vi "GetAttributes.vi"(0 "ClassReaderGOOP300 in":refnum<class "ClassReaderGOOP300.lvclass">, 1 "OnlyGetReference":bool, 5 "error in (no error)":errorcluster) -> (14 "ClassReaderGOOP300 out":refnum<class "ClassReaderGOOP300.lvclass">, 15 "ObjectAttributes":T1[](array[typedef])=[{"name"="MyU8", "type"=enum."UINT8", "dimension"=0, "typeName"="", "typePath"=path "", "visibility"=enum."Protected"}, {"name"="MyStrArray", "type"=enum."STRING", "dimension"=1, "typeName"="", "typePath"=path "", "visibility"=enum."Protected"}], 16 "ClassAttributes":T1[](array[typedef])=[{"name"="MyU8", "type"=enum."UINT8", "dimension"=0, "typeName"="", "typePath"=path "", "visibility"=enum."Protected"}, {"name"="MyStrArray", "type"=enum."STRING", "dimension"=1, "typeName"="", "typePath"=path "", "visibility"=enum."Protected"}], 17 "ObjectAttributeReference":refnum<vi>, 18 "ClassAttributeReference":refnum<vi>, 19 "error out":errorcluster)   [LabVIEW 2012, in "ClassReaderGOOP300.lvclass"]
uses:
  <resource>/Framework/Providers/Open_GDS/ClassProviders/Provider_EndevoGOOP300/ClassReaderGOOP300_class/ClassReaderGOOP300.lvclass
  <resource>/Framework/Providers/Open_GDS/UML/ReversedEngineering/ReversedEngineering AttributeInfoType.ctl
  <resource>/Framework/Providers/Open_GDS/ClassProviders/Common/CommonVIs/CommonVIs_AttributeDataType.ctl
  <resource>/Framework/Providers/Open_GDS/UML/UMLEditor/UMLEditor_VisibilityType.ctl
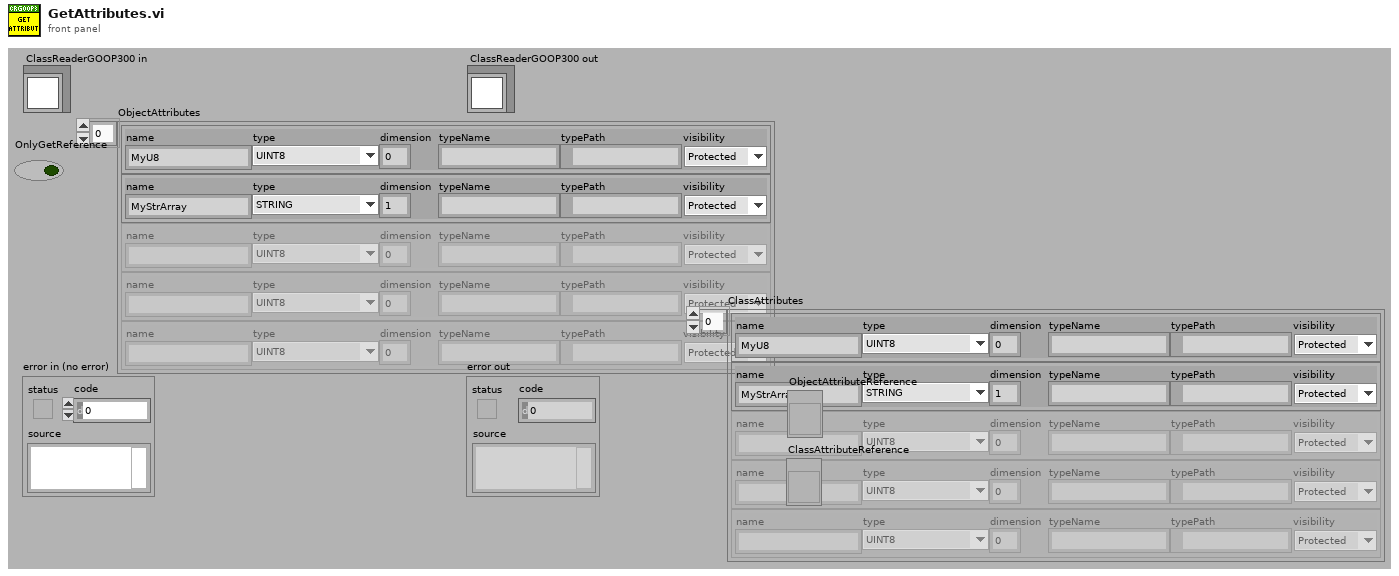
[diagram p1: front panel]
types:
  T1 = typedef "ReversedEngineering AttributeInfoType.ctl" = cluster{"name":string, "type":T2, "dimension":i32, "typeName":string, "typePath":path, "visibility":T3}
  T2 = typedef "CommonVIs_AttributeDataType.ctl" = enum16{"UINT8", "INT8", "UINT16", "INT16", "UINT32", "INT32", "UINT64", "INT64", "SGL", "DBL", "EXT", "CSG", "CDB", "CXT", "TimeStamp", "STRING", "PATH", "BOOL", "ENUM", "RefNum", "VIRefNum", "LabVIEW Class", "Cluster", "Variant", "TypeDef", "Waveform", "LabVIEW Object", "Other", "void"}
  T3 = typedef "UMLEditor_VisibilityType.ctl" = enum16{"Public", "Private", "Protected"}
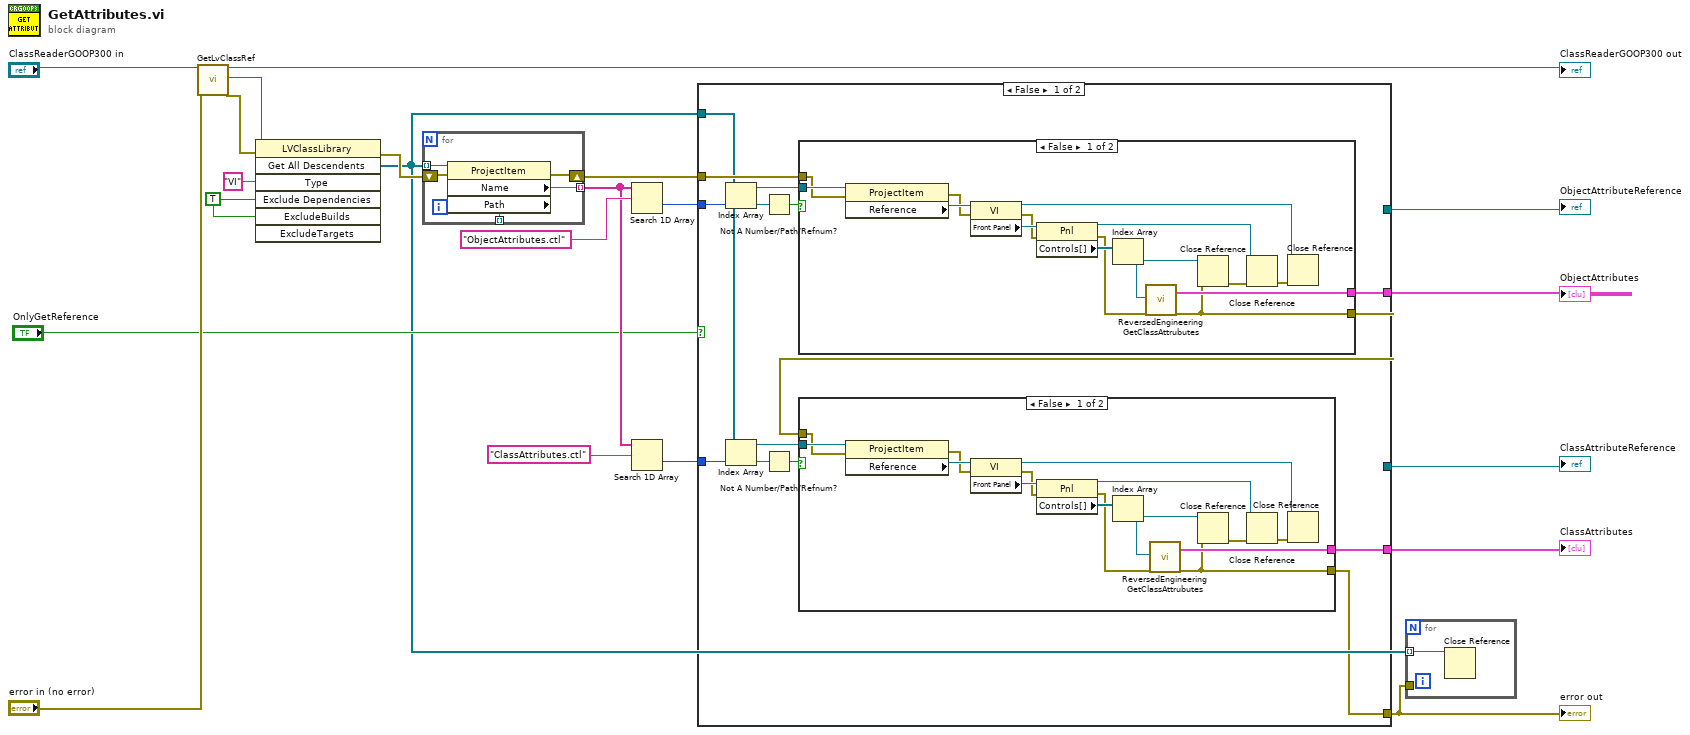
[diagram p0: block diagram]
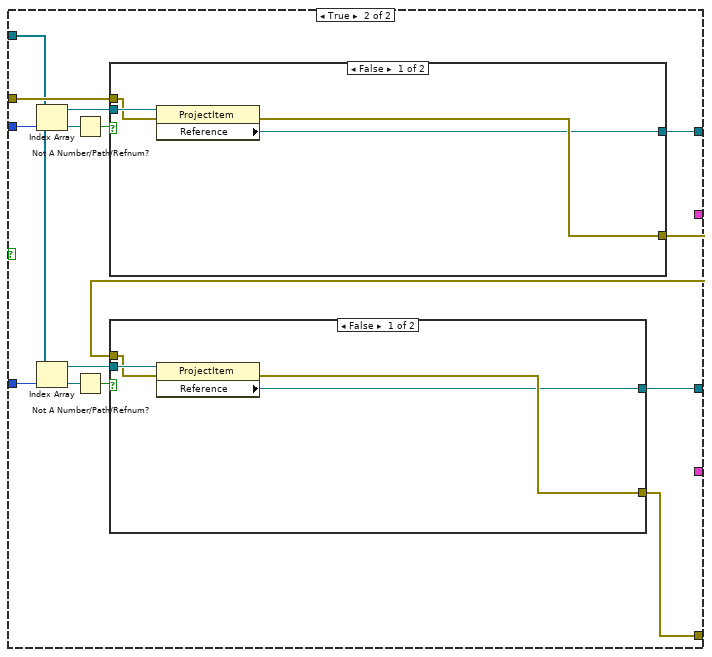
[diagram p4: hidden frame]
diagram:
  w2 = TRUE ("ExcludeDependencies")
  n1 = call-dynamic "GetLvClassRef.vi"("ClassReaderNative in"="ClassReaderGOOP300 in", "error in (no error)"="error in (no error)") -> ("ClassReaderNative out"=→"ClassReaderGOOP300 out":refnum<class "ClassReaderGOOP300.lvclass">, "LvClassRef"=w17:refnum<vi>, "error out"=w14:errorcluster)  [unwired: 15 in]
  n2 = invoke class="LVClassLibrary" method="Get All Descendents"(reference=w17, error in=w14, "Type"="VI", "Exclude Dependencies"=w2, "ExcludeBuilds"=w2) -> (error out=w15:errorcluster, "All Descendents"=w1:refnum<vi>[])  [unwired: 2 in, 5 out]
  n3 = for {
    tunnel: w1 -> [w26] mode=indexing
    tunnel: [w25] -> w11 mode=indexing
    shift-right: [w23] -> w12
    shift-left: w15 -> [w24]
    tunnel: [w22] -> _ mode=indexing
    n4 = property class="ProjectItem"(reference=w26, error in=w24) -> (error out=w23:errorcluster, "Name"=w25:string, "Path"=w22:path)  [unwired: 1 out]
  }
  n5 = Search 1D Array(1D array=w11, element="ObjectAttributes.ctl" ("string")) -> (index of element=w8:i32)  [unwired: 1 in]
  n6 = Search 1D Array(1D array=w11, element="ClassAttributes.ctl" ("string")) -> (index of element=w7:i32)  [unwired: 1 in]
  n7 = case shown="False" "OnlyGetReference" {
    tunnel: [w38 _] -> w19
    tunnel: w12 -> [w36 w81]
    tunnel: [w31 _] -> w9
    tunnel: [w30 w76] -> w3
    tunnel: w1 -> [w29 w75]
    tunnel: w8 -> [w28 w74]
    tunnel: w7 -> [w27 w73]
    tunnel: [_ w72] -> w5
    tunnel: [_ w71] -> w4
    frame False {
      n8 = Index Array(array=w29, index=w28) -> (element=w37:refnum<vi>)
      n9 = Index Array(array=w29, index=w27) -> (element=w33:refnum<vi>)
      n10 = Not A Number/Path/Refnum?(number/path/refnum=w37) -> (NaN/Path/Refnum?=w35:bool)
      n11 = Not A Number/Path/Refnum?(number/path/refnum=w33) -> (NaN/Path/Refnum?=w34:bool)
      n12 = case shown="False" w35 {
        tunnel: [w69 _] -> w38
        tunnel: w37 -> [w68 _]
        tunnel: w36 -> [w62 w70]
        tunnel: [w58 w70] -> w32
        frame False {
          n13 = property class="ProjectItem"(reference=w68, error in=w62) -> (error out=w63:errorcluster, "Reference"=w64:refnum<vi>)  [unwired: 1 out]
          n14 = property class="VI"(reference=w64, error in=w63) -> (reference out=w55:refnum<vi>, error out=w66:errorcluster, "Front Panel"=w67:refnum<vi>)
          n15 = property class="Pnl"(reference=w67, error in=w66) -> (reference out=w57:refnum<vi>, error out=w61:errorcluster, "Controls[]"=w65:refnum<vi>[])
          n16 = Index Array(array=w65) -> (element=w60:refnum<vi>)  [unwired: 1 in]
          n17 = call <resource>:"ReversedEngineering GetClassAttrubutes.vi"("CtlRefnum"=w60, "error in (no error)"=w61) -> ("attributeInfo"=w69:T1[], "error out"=w58:errorcluster)  [unwired: 15 in, 1 out]
          n18 = Close Reference(reference=w60, error in (no error)=w58) -> (error out=w59:errorcluster)
          n19 = Close Reference(reference=w57, error in (no error)=w59) -> (error out=w56:errorcluster)
          n20 = Close Reference(reference=w55, error in (no error)=w56) -> ()  [unwired: 1 out]
        }
        frame True {
        }
      }
      n21 = case shown="False" w34 {
        tunnel: [w53 _] -> w31
        tunnel: w33 -> [w52 _]
        tunnel: w32 -> [w46 w54]
        tunnel: [w41 w54] -> w30
        frame False {
          n22 = property class="ProjectItem"(reference=w52, error in=w46) -> (error out=w47:errorcluster, "Reference"=w48:refnum<vi>)  [unwired: 1 out]
          n23 = property class="VI"(reference=w48, error in=w47) -> (reference out=w39:refnum<vi>, error out=w50:errorcluster, "Front Panel"=w51:refnum<vi>)
          n24 = property class="Pnl"(reference=w51, error in=w50) -> (reference out=w40:refnum<vi>, error out=w45:errorcluster, "Controls[]"=w49:refnum<vi>[])
          n25 = Index Array(array=w49) -> (element=w42:refnum<vi>)  [unwired: 1 in]
          n26 = call <resource>:"ReversedEngineering GetClassAttrubutes.vi"("CtlRefnum"=w42, "error in (no error)"=w45) -> ("attributeInfo"=w53:T1[], "error out"=w41:errorcluster)  [unwired: 15 in, 1 out]
          n27 = Close Reference(reference=w42, error in (no error)=w41) -> (error out=w43:errorcluster)
          n28 = Close Reference(reference=w40, error in (no error)=w43) -> (error out=w44:errorcluster)
          n29 = Close Reference(reference=w39, error in (no error)=w44) -> ()  [unwired: 1 out]
        }
        frame True {
        }
      }
    }
    frame True {
      n30 = Index Array(array=w75, index=w74) -> (element=w82:refnum<vi>)
      n31 = Index Array(array=w75, index=w73) -> (element=w78:refnum<vi>)
      n32 = Not A Number/Path/Refnum?(number/path/refnum=w82) -> (NaN/Path/Refnum?=w80:bool)
      n33 = Not A Number/Path/Refnum?(number/path/refnum=w78) -> (NaN/Path/Refnum?=w79:bool)
      n34 = case shown="False" w80 {
        tunnel: w82 -> [w91 _]
        tunnel: w81 -> [w90 w92]
        tunnel: [w89 w92] -> w77
        tunnel: [w88 _] -> w72
        frame False {
          n35 = property class="ProjectItem"(reference=w91, error in=w90) -> (error out=w89:errorcluster, "Reference"=w88:refnum<vi>)  [unwired: 1 out]
        }
        frame True {
        }
      }
      n36 = case shown="False" w79 {
        tunnel: w78 -> [w86 _]
        tunnel: w77 -> [w85 w87]
        tunnel: [w84 w87] -> w76
        tunnel: [w83 _] -> w71
        frame False {
          n37 = property class="ProjectItem"(reference=w86, error in=w85) -> (error out=w84:errorcluster, "Reference"=w83:refnum<vi>)  [unwired: 1 out]
        }
        frame True {
        }
      }
    }
  }
  "ObjectAttributes" <- w19
  "ClassAttributes" <- w9
  "error out" <- w3
  "ClassAttributeReference" <- w4
  "ObjectAttributeReference" <- w5
  n38 = for {
    tunnel: w3 -> [_]
    tunnel: w1 -> [w93] mode=indexing
    n39 = Close Reference(reference=w93) -> ()  [unwired: 1 in, 1 out]
  }
